vi "Beta 2.3.2.vi"() -> ()   [LabVIEW 2011]
uses:
  <vilib>/vision/NI_Vision_Development_Module.lvlib
panel:
  in  "Structuring Element":dbl[][](array[numeric])=[[0.0, 1.0, 0.0], [1.0, 1.0, 1.0], [0.0, 1.0, 0.0]]
  in  "Morphology":u16(ring) items=["(none)", "AutoM", "Close", "Dilate", "Erode", "Gradient", "Gradient out", "Gradient in", "Open", "Thick", "Thin"]
  in  "Generate":bool
  in  "Look for":enum16{"Bright Objects", "Dark Objects"}(ring)
  in  "Method":T1(ring)=enum."Inter-class Variance"
  out "Binary":T2(plugin-control)
  out "Threshold Range":cluster{"Lower value":sgl, "Upper value":sgl}={"Lower value"=128.0, "Upper value"=255.0} {"Upper value" format="%.2f"; "Lower value" format="%.2f"}
  in  "Stop":bool
  in  "Browse":bool
  out "XY Graph":cluster{dbl[], dbl[]}(graph)
  out "Original Image":T2(plugin-control)
  out "Path to Image":path
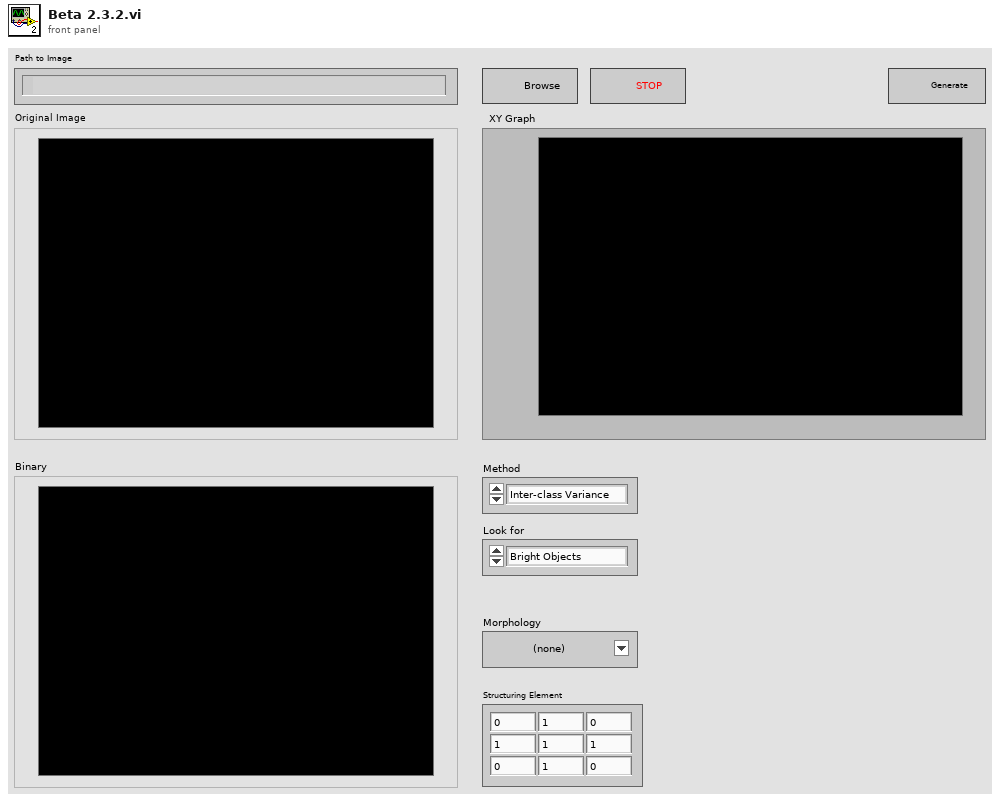
[diagram p1: front panel]
types:
  T1 = enum16{"Clustering", "Entropy", "Metric", "Moments", "Inter-class Variance"}
  T2 = typedef "IMAQ Image.ctl" = refnum<image>
  T3 = typedef "Image Type" = u32
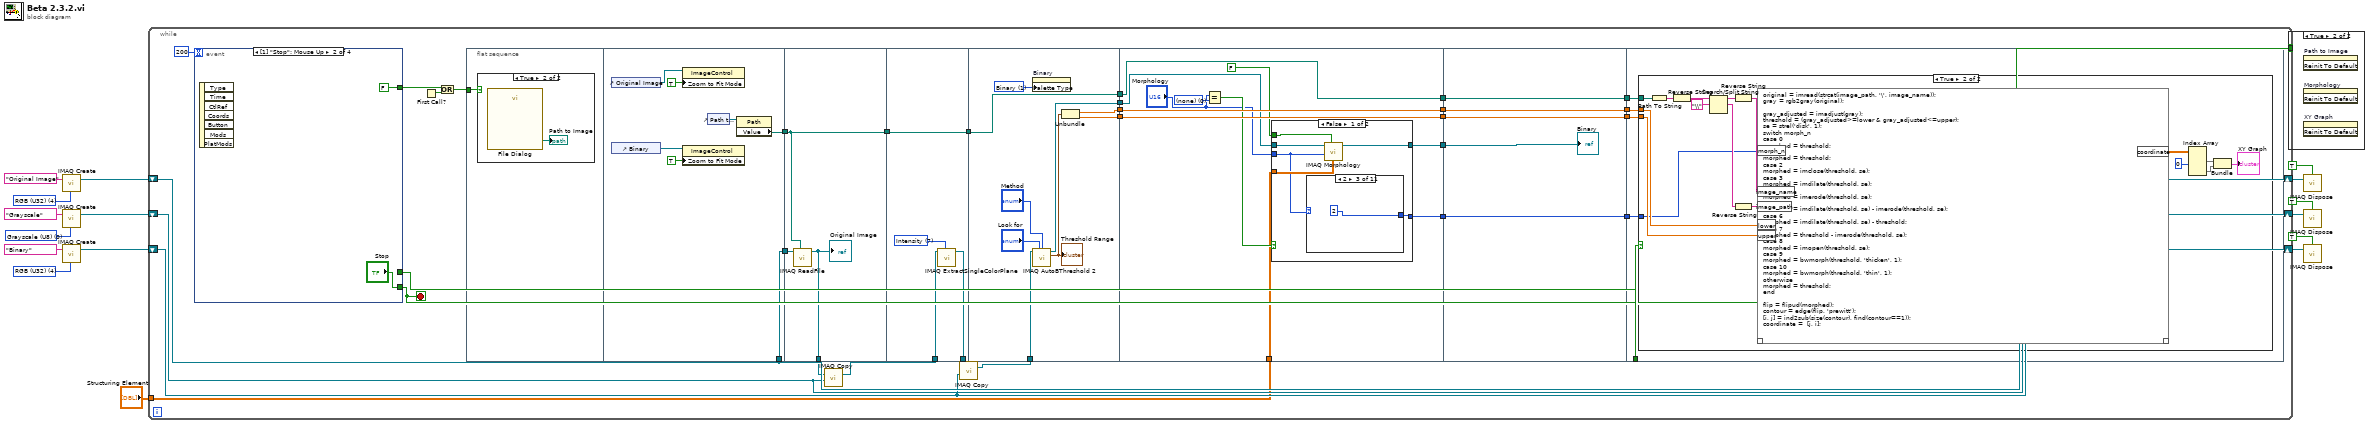
[diagram p0: block diagram]
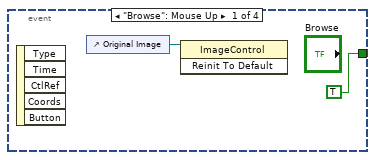
[diagram p3: hidden frame]
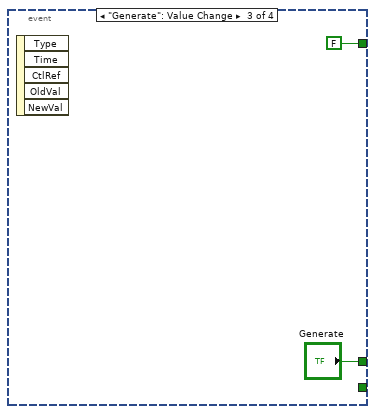
[diagram p4: hidden frame]
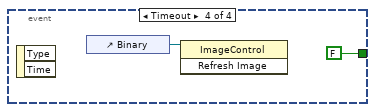
[diagram p5: hidden frame]
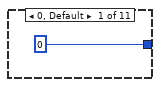
[diagram p7: hidden frame]
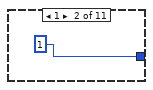
[diagram p8: hidden frame]
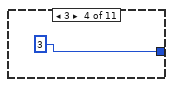
[diagram p9: hidden frame]
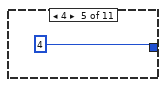
[diagram p10: hidden frame]
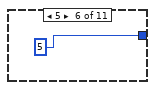
[diagram p11: hidden frame]
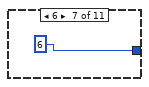
[diagram p12: hidden frame]
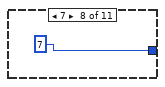
[diagram p13: hidden frame]
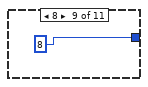
[diagram p14: hidden frame]
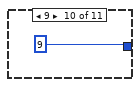
[diagram p15: hidden frame]
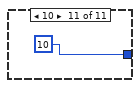
[diagram p16: hidden frame]
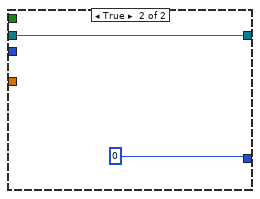
[diagram p17: hidden frame]
diagram:
  w5 = T3 4 items=["Grayscale (U8)", "Grayscale (I16)", "Grayscale (SGL)", "Complex (CSG)", "RGB (U32)", "HSL (U32)", "RGB (U64)", "Grayscale (U16)"] ("Image Type")
  w11 = T3 0 items=["Grayscale (U8)", "Grayscale (I16)", "Grayscale (SGL)", "Complex (CSG)", "RGB (U32)", "HSL (U32)", "RGB (U64)", "Grayscale (U16)"] ("Image Type")
  w16 = T3 4 items=["Grayscale (U8)", "Grayscale (I16)", "Grayscale (SGL)", "Complex (CSG)", "RGB (U32)", "HSL (U32)", "RGB (U64)", "Grayscale (U16)"] ("Image Type")
  n1 = call "IMAQ Create"("Image Name"="Original Image", "Image Type"=w16) -> ("New Image"=w15:T2)  [unwired: 3 in, 1 out]
  n2 = call "IMAQ Create"("Image Name"="Grayscale", "Image Type"=w11) -> ("New Image"=w10:T2)  [unwired: 3 in, 1 out]
  n3 = call "IMAQ Create"("Image Name"="Binary", "Image Type"=w5) -> ("New Image"=w2:T2)  [unwired: 3 in, 1 out]
  n4 = while {
    shift-right: [w43] -> w14
    shift-left: w15 -> [w43]
    tunnel: [w21] -> w13
    shift-right: [w37] -> w8
    shift-left: w10 -> [w37]
    shift-right: [w31] -> w3
    shift-left: w2 -> [w31]
    tunnel: "Structuring Element" -> [w20]
    stop <- w21 stop-if-true
    n5 = event shown="[1] \"Stop\": Mouse Up" {
      selector: _ -> [_ _ _ _]
      dyn-events: _ -> [_ _ _ _]
      timeout: 200 -> [_ _ _ _]
      tunnel: [TRUE FALSE FALSE FALSE] -> w47
      tunnel: [_ "Stop" _ _] -> w21
      tunnel: [_ _ "Generate" _] -> w36
      event "Browse": Mouse Up {
        n6 = event-data() -> ()  [unwired: 1 in, 5 out]
        n7 = control-ref of="Original Image"() -> (w50:refnum<vi>)
        n8 = invoke class="ImageControl" method="Reinit To Default"(reference=w50) -> ()  [unwired: 2 in, 3 out]
      }
      event "Stop": Mouse Up {
        n9 = event-data() -> ()  [unwired: 1 in, 7 out]
      }
      event "Generate": Value Change {
        n10 = event-data() -> ()  [unwired: 1 in, 5 out]
      }
      event Timeout {
        n11 = event-data() -> ()  [unwired: 1 in, 2 out]
        n12 = control-ref of="Binary"() -> (w56:refnum<vi>)
        n13 = invoke class="ImageControl" method="Refresh Image"(reference=w56) -> ()  [unwired: 2 in, 3 out]
      }
    }
    n14 = First Call?() -> (First Call?: T/F=w46:bool)
    n15 = Or(x=w47, y=w46) -> (x .or. y?=w45:bool)
    n16 = flat-sequence {
      tunnel: w45 -> [w57]
      tunnel: [w61] -> w48
      tunnel: [w62] -> w44
      tunnel: w43 -> [w61]
      tunnel: w48 -> [w67]
      tunnel: w44 -> [w68]
      tunnel: [w68] -> w42
      tunnel: [w66] -> w39
      tunnel: w42 -> [w72]
      tunnel: [w72] -> w41
      tunnel: w38 -> [w70]
      tunnel: [w69] -> w32
      tunnel: w41 -> [w81]
      tunnel: [w81] -> w29
      tunnel: [w80] -> w27
      tunnel: [w75] -> w26
      tunnel: [w74] -> w24
      tunnel: w33 -> [w73]
      tunnel: w29 -> [w92]
      tunnel: [w92] -> w28
      tunnel: w27 -> [w89]
      tunnel: w26 -> [w91]
      tunnel: [w91] -> w25
      tunnel: w24 -> [w90]
      tunnel: [w90] -> w23
      tunnel: [w88] -> w22
      tunnel: w20 -> [w83]
      tunnel: [w82] -> w19
      tunnel: w28 -> [w116]
      tunnel: [w116] -> w40
      tunnel: [w115] -> w35
      tunnel: w25 -> [w115]
      tunnel: [w114] -> w34
      tunnel: w23 -> [w114]
      tunnel: w22 -> [w113]
      tunnel: w19 -> [w112]
      tunnel: [w112] -> w18
      tunnel: w40 -> [w121]
      tunnel: w36 -> [w120]
      tunnel: w35 -> [w119]
      tunnel: w34 -> [w118]
      tunnel: w18 -> [w117]
      frame #0 {
        n17 = case shown="True" w57 {
          frame False {
          }
          frame True {
            n18 = call "File Dialog"() -> ("selected path"=→"Path to Image":path)  [unwired: 12 in, 3 out]
          }
        }
      }
      frame #1 {
        n19 = control-ref of="Original Image"() -> (w65:refnum<vi>)
        n20 = control-ref of="Binary"() -> (w60:refnum<vi>)
        n21 = property class="ImageControl"(reference=w65, "Zoom to Fit Mode"=TRUE) -> ()  [unwired: 1 in, 2 out]
        n22 = property class="ImageControl"(reference=w60, "Zoom to Fit Mode"=TRUE) -> ()  [unwired: 1 in, 2 out]
        n23 = control-ref of="Path to Image"() -> (w63:refnum<vi>)
        n24 = property class="Path"(reference=w63) -> ("Value"=w62:path)  [unwired: 1 in, 2 out]
      }
      frame #2 {
        n25 = call "IMAQ ReadFile"("File Path"=w68, "Image"=w67) -> ("Image Out"=w66:T2)  [unwired: 5 in, 4 out]
        "Original Image" <- w66
      }
      frame #3 {
        w71 = 7 items=["Red", "Green", "Blue", "Hue", "Saturation", "Luminance", "Value", "Intensity"] ("Color Plane")
        n26 = call "IMAQ ExtractSingleColorPlane"("Color Plane"=w71, "Image Src"=w70) -> ("Image Dst Out"=w69:T2)  [unwired: 8 in, 1 out]
      }
      frame #4 {
        w79 = u32 1 items=["Grayscale", "Binary", "Gradient", "Rainbow", "Temperature", "User Defined"] ("Palette")
        n27 = property on="Binary" class="ImageControl"("Palette Type"=w79) -> ()  [unwired: 2 in, 2 out]
        n28 = call "IMAQ AutoBThreshold 2"("Image Src"=w73, "Look For (Bright Objects)"="Look for", "Method (clustering)"="Method") -> ("Image Dst Out"=w80:T2, "Threshold Range Out"=w76:cluster{"Lower value":sgl, "Upper value":sgl})  [unwired: 10 in, 1 out]
        "Threshold Range" <- w76
        n29 = Unbundle(w76) -> ("Lower value"=w75:sgl, "Upper value"=w74:sgl)
      }
      frame #5 {
        w86 = u16 0 items=["(none)"]
        n30 = Equal?(x="Morphology", y=w86) -> (x = y?=w85:bool)
        n31 = case shown="False" w85 {
          tunnel: w89 -> [w96 w111]
          tunnel: [w97 w111] -> w88
          tunnel: FALSE -> [w98 _]
          tunnel: "Morphology" -> [w94 _]
          tunnel: w83 -> [w95 _]
          tunnel: [w93 0] -> w82
          frame False {
            n32 = case shown="2" w94 {
              tunnel: [0 1 2 3 4 5 6 7 8 9 10] -> w93
              frame 0, Default {
              }
              frame 1 {
              }
              frame 2 {
              }
              frame 3 {
              }
              frame 4 {
              }
              frame 5 {
              }
              frame 6 {
              }
              frame 7 {
              }
              frame 8 {
              }
              frame 9 {
              }
              frame 10 {
              }
            }
            n33 = call "IMAQ Morphology"("Structuring Element"=w95, "Square/Hexa (Square)"=w98, "Operation"=w94, "Image Src"=w96) -> ("Image Dst Out"=w97:T2)  [unwired: 6 in, 1 out]
          }
          frame True {
          }
        }
      }
      frame #6 {
        "Binary" <- w113
      }
      frame #7 {
        n34 = case shown="True" w120 {
          tunnel: w121 -> [_ w137]
          tunnel: w119 -> [_ w124]
          tunnel: w118 -> [_ w123]
          tunnel: w117 -> [_ w122]
          frame False {
          }
          frame True {
            n35 = Path To String(path=w137) -> (string=w136:string)
            n36 = Reverse String(1:w136) -> (0:w135:string)
            n37 = Search/Split String(string=w135, search string/char (-)="\\") -> (substring before match=w133:string, match + rest of string=w132:string)  [unwired: 1 in, 1 out]
            n38 = Reverse String(1:w133) -> (0:w131:string)
            n39 = Reverse String(1:w132) -> (0:w130:string)
            n40 = script code="original = imread(strcat(image_path, '\\', image_name));\ngray = rgb2gray(original);\n\ngray_adjusted = imadjust(gray);\nthreshold = (gray_adjusted>=lower & gray_adjusted<=upper);\nse = strel('disk', 1);\nswitch morph_n\ncase 0\nmorphed = threshold;\ncase 1\nmorphed = threshold;\ncase 2\nmorphed = imclose(threshold, se);\ncase 3\nmorphed = imdilate(threshold, se);\ncase 4\nmorphed = imerode(threshold, se);\ncase 5\nmorphed = imdilate(threshold, se) - imerode(threshold, se);\ncase 6\nmorphed = imdilate(threshold, se) - threshold;\ncase 7\nmorphed = threshold - imerode(threshold, se);\ncase 8\nmorphed = imopen(threshold, se);\ncase 9\nmorphed = bwmorph(threshold, 'thicken', 1);\ncase 10\nmorphed = bwmorph(threshold, 'thin', 1);\notherwise\nmorphed = threshold;\nend\n\nflip = flipud(morphed);\ncontour = edge(flip, 'prewitt');\n[i, j] = ind2sub(size(contour), find(contour==1));\ncoordinate =  [j, i];"("image_name"=w131, "image_path"=w130, "lower"=w124, "upper"=w123, "morph_n"=w122) -> ("coordinate"=w129:dbl[][])  [unwired: 1 in, 1 out]
            n41 = Index Array(array=w129, index (col) #1=0 ("disabled index (col)")) -> (element #1=w128:dbl[], element #2=w127:dbl[])  [unwired: 3 in]
            n42 = Bundle(w128, w127) -> (→"XY Graph":cluster{dbl[], dbl[]})  [unwired: 1 in]
          }
        }
      }
    }
    n43 = call "IMAQ Copy"("Image Dst"=w37, "Image Src"=w39) -> ("Image Dst Out"=w38:T2)  [unwired: 4 in, 1 out]
    n44 = call "IMAQ Copy"("Image Dst"=w31, "Image Src"=w32) -> ("Image Dst Out"=w33:T2)  [unwired: 4 in, 1 out]
  }
  n45 = case shown="True" w13 {
    frame False {
    }
    frame True {
      n46 = invoke on="Path to Image" class="Path" method="Reinit To Default"() -> ()  [unwired: 3 in, 3 out]
      n47 = invoke on="Morphology" class="Ring (strict)" method="Reinit To Default"() -> ()  [unwired: 3 in, 3 out]
      n48 = invoke on="XY Graph" class="XYGraph (strict)" method="Reinit To Default"() -> ()  [unwired: 3 in, 3 out]
    }
  }
  n49 = call "IMAQ Dispose"("All Images? (No)"=TRUE, "Image"=w14) -> ()  [unwired: 4 in, 1 out]
  n50 = call "IMAQ Dispose"("All Images? (No)"=TRUE, "Image"=w8) -> ()  [unwired: 4 in, 1 out]
  n51 = call "IMAQ Dispose"("All Images? (No)"=TRUE, "Image"=w3) -> ()  [unwired: 4 in, 1 out]
